vi "buildPath.vi"(11 "Path Name List":string[](array[string])) -> (3 "New Path":path)   [LabVIEW 2016]
doc: "Built the path."
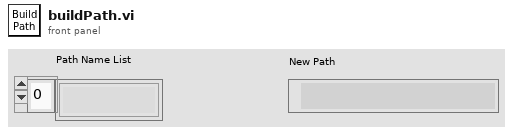
[diagram p1: front panel]
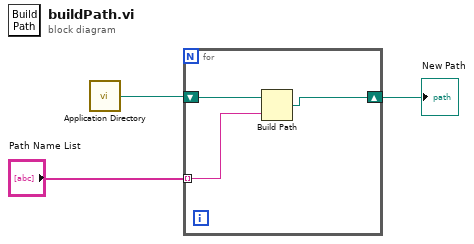
[diagram p0: block diagram]
diagram:
  n1 = call <vilib>:"Application Directory.vi"() -> ("Application Directory"=w1:path)
  n2 = for {
    tunnel: "Path Name List" -> [w6] mode=indexing
    shift-right: [w4] -> w2
    shift-left: w1 -> [w5]
    n3 = Build Path(base path=w5, name or relative path=w6) -> (appended path=w4:path)
  }
  "New Path" <- w2
